vi "Get Headers.vi"(8 "error in (no error)":errorcluster, 11 "SLL Table in":refnum<class "SLL Table.lvclass">) -> (0 "error out":errorcluster, 2 "Headers[]":string[](array[string]), 3 "SLL Table out":refnum<class "SLL Table.lvclass">)   [LabVIEW 2019, in "SLL Table.lvclass"]
doc: "Returns the available headers of the table."
uses:
  SLL Table.lvclass
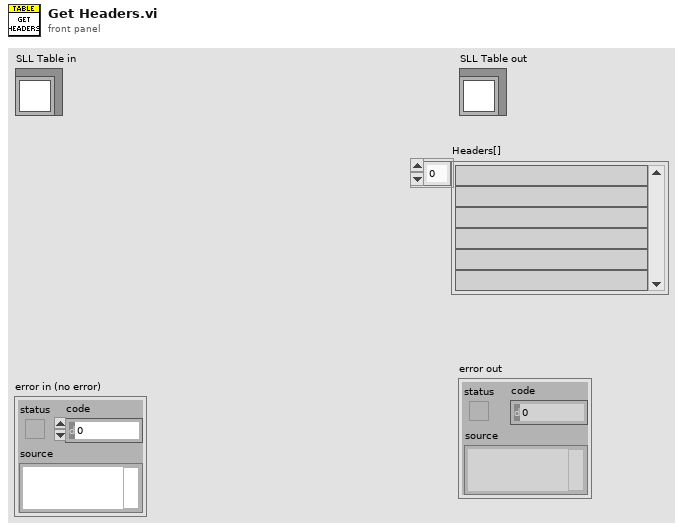
[diagram p1: front panel]
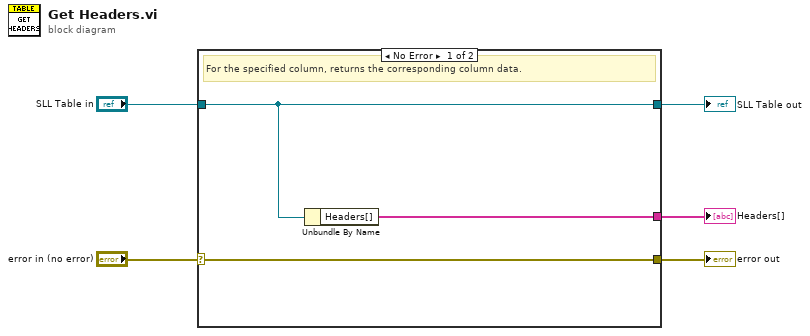
[diagram p0: block diagram]
diagram:
  n1 = case shown="No Error" "error in (no error)" {
    selector: "error in (no error)" -> [w8 w10]
    tunnel: [w8 w10] -> w4
    tunnel: [w7 w9] -> w2
    tunnel: "SLL Table in" -> [w7 w9]
    tunnel: [w6 _] -> w1
    frame No Error {
      # "For the specified column, returns the corresponding column data."
      n2 = Unbundle By Name(w7) -> ("Headers[]"=w6:string[])
    }
    frame Error {
    }
  }
  "error out" <- w4
  "SLL Table out" <- w2
  "Headers[]" <- w1
